vi "Setup Statically-Linked subWorkers.vi"(8 "error in":errorcluster, 11 "Host NI 9205 Demo in":refnum<class "Host NI 9205 Demo.lvclass">) -> (0 "error out":errorcluster, 3 "Host NI 9205 Demo out":refnum<class "Host NI 9205 Demo.lvclass">)   [LabVIEW 2017, in "Host NI 9205 Demo.lvclass"]
doc: "This VI performs a setup of all the statically-linked subWorkers that belong to the Worker that owns this VI. This VI must be called <b>before</b> any statically-linked subWorkers are called."
uses:
  Host NI 9205 Demo.lvclass
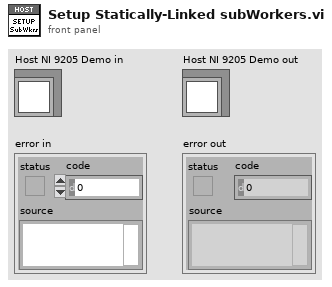
[diagram p1: front panel]
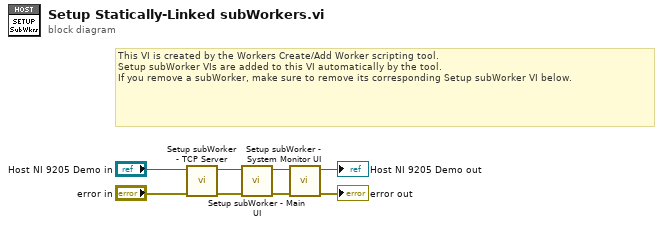
[diagram p0: block diagram]
diagram:
  # "This VI is created by the Workers Create/Add Worker scripting tool.\nSetup subWorker VIs are added to this VI automatically by the tool.\nIf you remove a subWorker, make sure to remove its corresponding Setup subWorker VI below."
  n1 = call "Setup subWorker - TCP Server.vi"("error in"="error in", "Host NI 9205 Demo in"="Host NI 9205 Demo in") -> ("error out"=w7:errorcluster, "Host NI 9205 Demo out"=w4:refnum<class "Host NI 9205 Demo.lvclass">)  [unwired: 8 in]
  n2 = call "Setup subWorker - Main UI.vi"("error in"=w7, "Host NI 9205 Demo in"=w4) -> ("error out"=w5:errorcluster, "Host NI 9205 Demo out"=w2:refnum<class "Host NI 9205 Demo.lvclass">)  [unwired: 8 in]
  n3 = call "Setup subWorker - System Monitor UI.vi"("error in"=w5, "Host NI 9205 Demo in"=w2) -> ("error out"=→"error out":errorcluster, "Host NI 9205 Demo out"=→"Host NI 9205 Demo out":refnum<class "Host NI 9205 Demo.lvclass">)  [unwired: 8 in]
